vi "Initialize Sequence.vi"(8 "error in (no error)":errorcluster, 10 "Current Time":dbl, 11 "Output Sequencer in":refnum<class "Output Sequencer.lvclass">) -> (0 "error out":errorcluster, 3 "Output Sequencer out":refnum<class "Output Sequencer.lvclass">)   [LabVIEW 2020, in "Output Sequencer.lvlib" / "Output Sequencer.lvclass"]
uses:
  Output Sequencer.lvclass
  Output Sequencer.lvclass/Output Sequencer.ctl
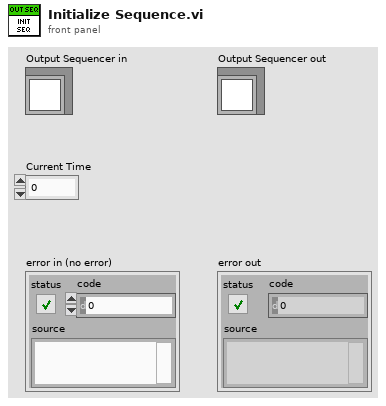
[diagram p1: front panel]
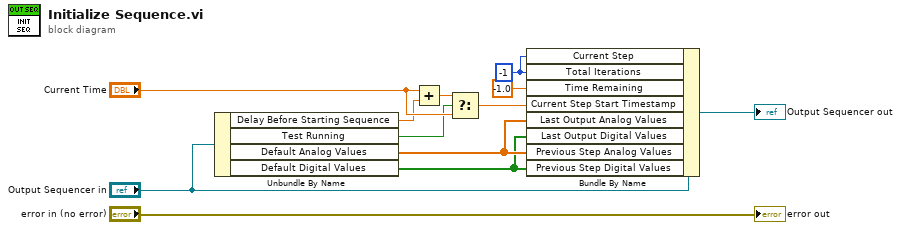
[diagram p0: block diagram]
diagram:
  w8 = -1 ("Total Iterations")
  n1 = Unbundle By Name("Output Sequencer in") -> ("Delay Before Starting Sequence"=w3:dbl, "Test Running"=w6:bool, "Default Analog Values"=w2:dbl[], "Default Digital Values"=w1:bool[])
  n2 = Add(x="Current Time", y=w3) -> (x+y=w7:dbl)
  n3 = Select(t=w7, s=w6, f="Current Time") -> (s? t:f=w4:dbl)
  n4 = Bundle By Name(cluster="Output Sequencer in", "Current Step"=w8, "Total Iterations"=w8, "Time Remaining"=-1.0, "Current Step Start Timestamp"=w4, "Last Output Analog Values"=w2, "Last Output Digital Values"=w1, "Previous Step Analog Values"=w2, "Previous Step Digital Values"=w1) -> (→"Output Sequencer out":refnum<class "Output Sequencer.lvclass">)
  "error out" <- "error in (no error)"
